vi "Write Store.vi"(8 "error in (no error)":errorcluster, 10 "Store Actor":refnum<class "VIStore.lvclass">, 11 "StoreUI in":refnum<class "StoreUI.lvclass">) -> (0 "error out":errorcluster, 3 "StoreUI out":refnum<class "StoreUI.lvclass">)   [LabVIEW 2015, in "StoreUI.lvlib" / "StoreUI.lvclass"]
uses:
  StoreUI.lvclass
  VI Store/VIStore Actor/VIStore.lvclass
  StoreUI.lvclass/StoreUI.ctl
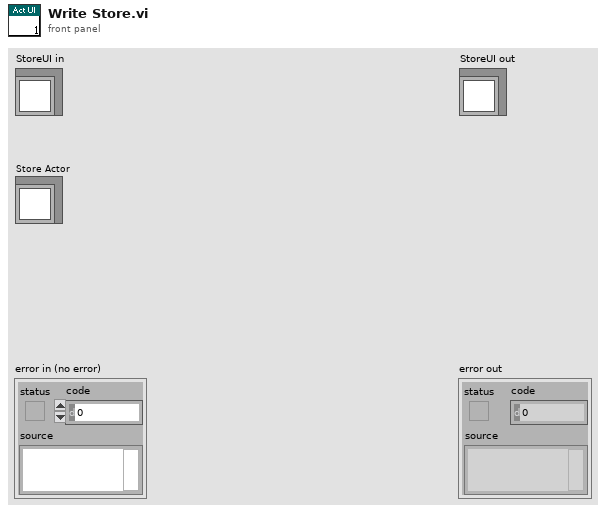
[diagram p1: front panel]
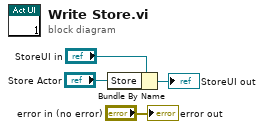
[diagram p0: block diagram]
diagram:
  n1 = Bundle By Name(cluster="StoreUI in", "Store"="Store Actor") -> (→"StoreUI out":refnum<class "StoreUI.lvclass">)
  "error out" <- "error in (no error)"
